vi "Perform Work.vi"(6 "Last request":bool, 8 "error in (no error)":errorcluster, 9 "Initialize":bool, 10 "Reply to":refnum<class "Result Reply Msg.lvclass">, 11 "Measure Object in":refnum<class "Worker.lvclass">) -> (0 "error out":errorcluster, 3 "Measure Object out":refnum<class "Worker.lvclass">)   [LabVIEW 2019, in "Worker.lvclass"]
uses:
  Worker.lvclass
  C:/GitHub/LabActor/Template Module/Template Module.lvclass
  C:/Program Files/National Instruments/LabVIEW 2019/vi.lib/ActorFramework/Actor/Actor.lvclass
  Template Module Messages/Result Reply Msg/Result Reply Msg.lvclass
  Worker.lvclass/Worker.ctl
  Template Module/Template Module.lvclass/Template Module.ctl
  NHMFL_Core/Libraries/Instruments/Results/Acquired Result/Acquired Result.lvclass/Acquired Result.ctl
  <vilib>/ActorFramework/Actor/Actor.lvclass/Actor.ctl
  <vilib>/ActorFramework/Message Enqueuer/Message Enqueuer.lvclass/Message Enqueuer.ctl
  Pulse Recorders/Pulse Recorder Messages/Wait for Data Msg/Wait for Result Msg.lvclass/Wait for Result Msg.ctl
  Write Done.vi
  NHMFL_Core/Libraries/Instruments/Results/Acquired Result/Read Final.vi
  Template Module/Read Reply to.vi
  Template Module/Read Name.vi
  NHMFL_Core/Libraries/Instruments/Results/Acquired Result/Write Sender.vi
  NHMFL_Core/Libraries/Instruments/Results/Acquired Result/Write Cycle count.vi
  Read Check again delay.vi
  Template Module/Write Reply to.vi
  Template Module/Read State.vi
  <vilib>/ActorFramework/Message Enqueuer/Init from Existing Queue.vi
  Pulse Recorders/Pulse Recorder Messages/Wait for Data Msg/Wait for Result Msg.lvclass
  C:/Program Files/National Instruments/LabVIEW 2019/vi.lib/ActorFramework/Message/Message.lvclass
  <vilib>/ActorFramework/Time-Delayed Send Message/Time-Delayed Send Message.vi
  <vilib>/ActorFramework/Message Enqueuer/Message Enqueuer.lvclass
  <vilib>/ActorFramework/Actor/Actor.lvclass
  NHMFL_Core/Libraries/Instruments/Results/Acquired Result/Acquired Result.lvclass
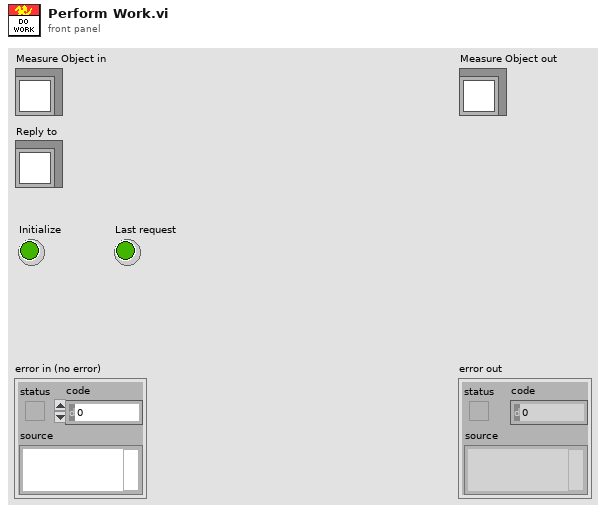
[diagram p1: front panel]
types:
  T1 = typedef "Worker State.ctl" = enum16{"Idle", "Starting", "Working", "Stopping"}
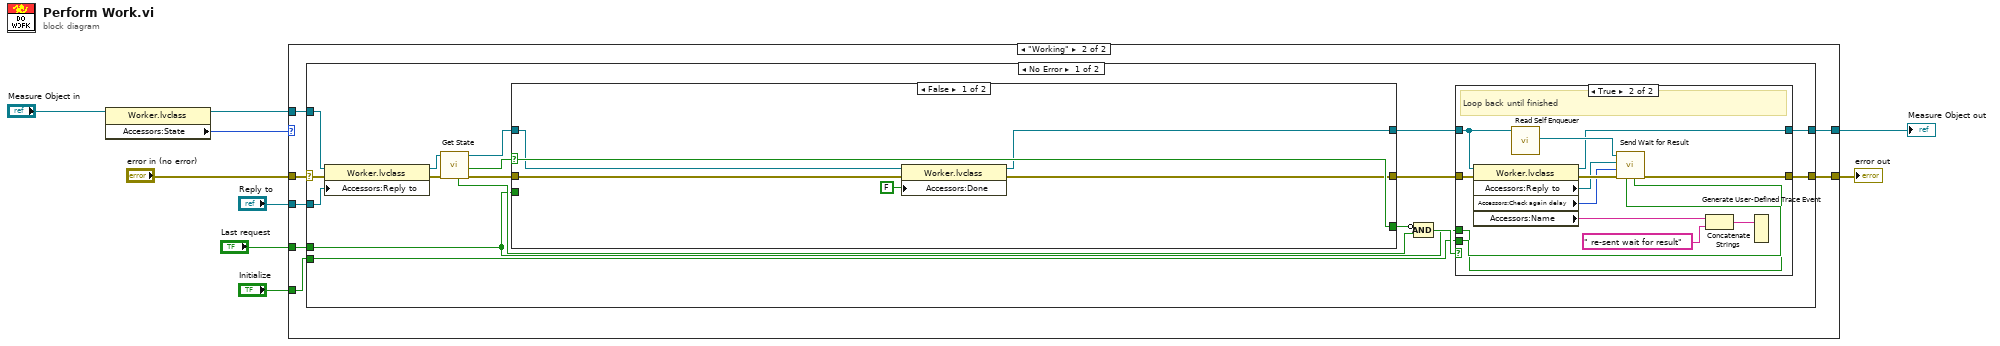
[diagram p0: block diagram]
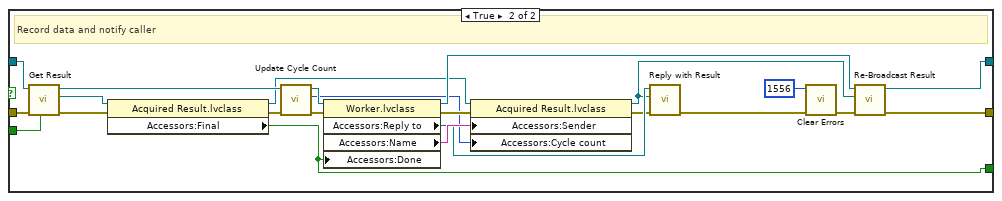
[diagram p4: hidden frame]
diagram:
  n1 = property class="Worker.lvclass"(reference="Measure Object in") -> (reference out=w4:refnum<class "Worker.lvclass">, "Accessors:State"=w3:T1)  [unwired: 1 in, 1 out]
  n2 = case shown="\"Working\"" w3 {
    tunnel: "error in (no error)" -> [w10 w18]
    tunnel: [w10 w17] -> w8
    tunnel: [w11 w16] -> w7
    tunnel: "Reply to" -> [_ w15]
    tunnel: w4 -> [w11 w14]
    tunnel: "Last request" -> [_ w13]
    tunnel: "Initialize" -> [_ w12]
    frame "Idle", Default {
    }
    frame "Working" {
      n3 = case shown="No Error" w18 {
        selector: w18 -> [w34 w81]
        tunnel: [w21 w81] -> w17
        tunnel: [w23 w80] -> w16
        tunnel: w15 -> [w35 _]
        tunnel: w14 -> [w33 w80]
        tunnel: w13 -> [w19 _]
        tunnel: w12 -> [w20 _]
        frame No Error {
          n4 = property class="Worker.lvclass"(reference=w33, error in=w34, "Accessors:Reply to"=w35) -> (reference out=w24:refnum<class "Worker.lvclass">, error out=w22:errorcluster)
          n5 = call-dynamic "Get State.vi"("error in (no error)"=w22, "Worker in"=w24) -> ("error out"=w31:errorcluster, "Result ready"=w32:bool, "Worker out"=w30:refnum<class "Worker.lvclass">, "Check again"=w28:bool)  [unwired: 5 in, 1 out]
          n6 = case shown="False" w32 {
            selector: w32 -> [w55 _]
            tunnel: w30 -> [w53 w79]
            tunnel: w31 -> [w56 w78]
            tunnel: [w54 w69] -> w26
            tunnel: [w52 w68] -> w25
            tunnel: [w55 w57] -> w29
            tunnel: w19 -> [_ w67]
            frame False {
              n7 = property class="Worker.lvclass"(reference=w53, error in=w56, "Accessors:Done"=FALSE ("Done")) -> (reference out=w52:refnum<class "Worker.lvclass">, error out=w54:errorcluster)
            }
            frame True {
              # "Record data and notify caller"
              n8 = call-dynamic "Get Result.vi"("Last request"=w67, "error in (no error)"=w78, "Worker in"=w79) -> ("error out"=w73:errorcluster, "Result"=w59:refnum<class "Acquired Result.lvclass">, "Worker out"=w65:refnum<class "Worker.lvclass">)  [unwired: 6 in]
              n9 = property class="Acquired Result.lvclass"(reference=w59, error in=w73) -> (reference out=w58:refnum<class "Acquired Result.lvclass">, error out=w60:errorcluster, "Accessors:Final"=w57:bool)
              n10 = call-dynamic "Update Cycle Count.vi"("error in (no error)"=w60, "Worker in"=w65) -> ("error out"=w66:errorcluster, "Cycle count out"=w63:i32, "Worker out"=w64:refnum<class "Worker.lvclass">)  [unwired: 7 in]
              n11 = property class="Worker.lvclass"(reference=w64, error in=w66, "Accessors:Done"=w57) -> (reference out=w72:refnum<class "Worker.lvclass">, error out=w77:errorcluster, "Accessors:Reply to"=w75:refnum<class "Result Reply Msg.lvclass">, "Accessors:Name"=w76:string)
              n12 = property class="Acquired Result.lvclass"(reference=w58, error in=w77, "Accessors:Sender"=w76, "Accessors:Cycle count"=w63) -> (reference out=w71:refnum<class "Acquired Result.lvclass">, error out=w74:errorcluster)
              n13 = call-dynamic "Reply with Result.vi"("error in (no error)"=w74, "Result"=w71, "Result Reply Msg in"=w75) -> ("error out"=w70:errorcluster)  [unwired: 7 in, 1 out]
              n14 = call <vilib>:"Clear Errors.vi"("error in (no error)"=w70, "specific error code to clear (0: all)"=1556) -> ("error out"=w62:errorcluster)  [unwired: 4 in, 1 out]
              n15 = call-dynamic "Re-Broadcast Result.vi"("error in (no error)"=w62, "Acquired Result.lvclass"=w71, "Measure Object in"=w72) -> ("error out"=w69:errorcluster, "Measure Object out"=w68:refnum<class "Worker.lvclass">)  [unwired: 7 in]
            }
          }
          n16 = Compound Arithmetic op=AND(invert w29, w28) -> (w27:bool)
          n17 = case shown="True" w27 {
            tunnel: w25 -> [w36 w48]
            tunnel: w26 -> [w37 w45]
            tunnel: [w37 w49] -> w21
            tunnel: [w36 w43] -> w23
            tunnel: w20 -> [_ w41]
            tunnel: w19 -> [_ w40]
            frame False {
            }
            frame True {
              # "Loop back until finished"
              n18 = property class="Worker.lvclass"(reference=w48, error in=w45) -> (reference out=w43:refnum<class "Worker.lvclass">, error out=w44:errorcluster, "Accessors:Reply to"=w38:refnum<class "Result Reply Msg.lvclass">, "Accessors:Check again delay"=w39:i32, "Accessors:Name"=w42:string)
              n19 = call <vilib>:"Read Self Enqueuer.vi"("Actor"=w48) -> ("Self Enqueuer"=w50:refnum<class "Message Enqueuer.lvclass">)  [unwired: 10 in]
              n20 = call "Send Wait for Result.vi"("Last request"=w40, "Initialize"=w41, "error in (no error)"=w44, "Milliseconds To Wait"=w39, "Reply to"=w38, "Message Enqueuer"=w50) -> ("error out"=w49:errorcluster)  [unwired: 3 in, 2 out]
              n21 = Concatenate Strings(w42, " re-sent wait for result" ("string")) -> (w46:string)
              n22 = Generate User-Defined Trace Event(2:w46) -> ()  [unwired: 1 in]
            }
          }
        }
        frame Error {
        }
      }
    }
  }
  "error out" <- w8
  "Measure Object out" <- w7
